vi "test TCX read (installed 71).vi"() -> ()   [LabVIEW 2011] (continued)
rees></Position><AltitudeMeters>71.275</AltitudeMeters><DistanceMeters>20043.990</DistanceMeters><Cadence>68</Cadence><Extensions><TPX xmlns=\"http://www.garmin.com/xmlschemas/ActivityExtension/v2\"><Watts>169</Watts></TPX></Extensions></Trackpoint><Trackpoint><Time>2008-03-03T23:21:45Z</Time><Position><LatitudeDegrees>35.876197</LatitudeDegrees><LongitudeDegrees>-78.946791</LongitudeDegrees></Position><AltitudeMeters>71.755</AltitudeMeters><DistanceMeters>20051.418</DistanceMeters><Cadence>67</Cadence><Extensions><TPX xmlns=\"http://www.garmin.com/xmlschemas/ActivityExtension/v2\"><Watts>175</Watts></TPX></Extensions></Trackpoint><Trackpoint><Time>2008-03-03T23:21:46Z</Time><Position><LatitudeDegrees>35.876203</LatitudeDegrees><LongitudeDegrees>-78.946872</LongitudeDegrees></Position><AltitudeMeters>72.236</AltitudeMeters><DistanceMeters>20058.742</DistanceMeters><Cadence>67</Cadence><Extensions><TPX xmlns=\"http://www.garmin.com/xmlschemas/ActivityExtension/v2\"><Watts>174</Watts></TPX></Extensions></Trackpoint><Trackpoint><Time>2008-03-03T23:21:47Z</Time><Position><LatitudeDegrees>35.876206</LatitudeDegrees><LongitudeDegrees>-78.946951</LongitudeDegrees></Position><AltitudeMeters>72.236</AltitudeMeters><DistanceMeters>20065.842</DistanceMeters><Cadence>65</Cadence><Extensions><TPX xmlns=\"http://www.garmin.com/xmlschemas/ActivityExtension/v2\"><Watts>166</Watts></TPX></Extensions></Trackpoint><Trackpoint><Time>2008-03-03T23:21:48Z</Time><Position><LatitudeDegrees>35.876207</LatitudeDegrees><LongitudeDegrees>-78.947027</LongitudeDegrees></Position><AltitudeMeters>72.236</AltitudeMeters><DistanceMeters>20072.709</DistanceMeters><Cadence>63</Cadence><Extensions><TPX xmlns=\"http://www.garmin.com/xmlschemas/ActivityExtension/v2\"><Watts>171</Watts></TPX></Extensions></Trackpoint><Trackpoint><Time>2008-03-03T23:21:49Z</Time><Position><LatitudeDegrees>35.876210</LatitudeDegrees><LongitudeDegrees>-78.947102</LongitudeDegrees></Position><AltitudeMeters>72.236</AltitudeMeters><DistanceMeters>20079.447</DistanceMeters><Cadence>62</Cadence><Extensions><TPX xmlns=\"http://www.garmin.com/xmlschemas/ActivityExtension/v2\"><Watts>177</Watts></TPX></Extensions></Trackpoint><Trackpoint><Time>2008-03-03T23:21:50Z</Time><Position><LatitudeDegrees>35.876215</LatitudeDegrees><LongitudeDegrees>-78.947175</LongitudeDegrees></Position><AltitudeMeters>72.717</AltitudeMeters><DistanceMeters>20086.098</DistanceMeters><Cadence>68</Cadence><Extensions><TPX xmlns=\"http://www.garmin.com/xmlschemas/ActivityExtension/v2\"><Watts>192</Watts></TPX></Extensions></Trackpoint><Trackpoint><Time>2008-03-03T23:21:51Z</Time><Position><LatitudeDegrees>35.876220</LatitudeDegrees><LongitudeDegrees>-78.947248</LongitudeDegrees></Position><AltitudeMeters>72.717</AltitudeMeters><DistanceMeters>20092.703</DistanceMeters><Cadence>68</Cadence><Extensions><TPX xmlns=\"http://www.garmin.com/xmlschemas/ActivityExtension/v2\"><Watts>200</Watts></TPX></Extensions></Trackpoint><Trackpoint><Time>2008-03-03T23:21:52Z</Time><Position><LatitudeDegrees>35.876223</LatitudeDegrees><LongitudeDegrees>-78.947321</LongitudeDegrees></Position><AltitudeMeters>73.198</AltitudeMeters><DistanceMeters>20099.342</DistanceMeters><Cadence>68</Cadence><Extensions><TPX xmlns=\"http://www.garmin.com/xmlschemas/ActivityExtension/v2\"><Watts>201</Watts></TPX></Extensions></Trackpoint><Trackpoint><Time>2008-03-03T23:21:53Z</Time><Position><LatitudeDegrees>35.876227</LatitudeDegrees><LongitudeDegrees>-78.947395</LongitudeDegrees></Position><AltitudeMeters>73.198</AltitudeMeters><DistanceMeters>20106.008</DistanceMeters><Cadence>67</Cadence><Extensions><TPX xmlns=\"http://www.garmin.com/xmlschemas/ActivityExtension/v2\"><Watts>197</Watts></TPX></Extensions></Trackpoint><Trackpoint><Time>2008-03-03T23:21:54Z</Time><Position><LatitudeDegrees>35.876231</LatitudeDegrees><LongitudeDegrees>-78.947468</LongitudeDegrees></Position><AltitudeMeters>73.198</AltitudeMeters><DistanceMeters>20112.586</DistanceMeters><Cadence>67</Cadence><Extensions><TPX xmlns=\"http://www.garmin.com/xmlschemas/ActivityExtension/v2\"><Watts>192</Watts></TPX></Extensions></Trackpoint><Trackpoint><Time>2008-03-03T23:21:55Z</Time><Position><LatitudeDegrees>35.876232</LatitudeDegrees><LongitudeDegrees>-78.947539</LongitudeDegrees></Position><AltitudeMeters>73.198</AltitudeMeters><DistanceMeters>20118.984</DistanceMeters><Cadence>66</Cadence><Extensions><TPX xmlns=\"http://www.garmin.com/xmlschemas/ActivityExtension/v2\"><Watts>180</Watts></TPX></Extensions></Trackpoint><Trackpoint><Time>2008-03-03T23:21:56Z</Time><Position><LatitudeDegrees>35.876232</LatitudeDegrees><LongitudeDegrees>-78.947610</LongitudeDegrees></Position><AltitudeMeters>73.678</AltitudeMeters><DistanceMeters>20125.402</DistanceMeters><Cadence>66</Cadence><Extensions><TPX xmlns=\"http://www.garmin.com/xmlschemas/ActivityExtension/v2\"><Watts>188</Watts></TPX></Extensions></Trackpoint><Trackpoint><Time>2008-03-03T23:21:57Z</Time><Position><LatitudeDegrees>35.876234</LatitudeDegrees><LongitudeDegrees>-78.947681</LongitudeDegrees></Position><AltitudeMeters>73.678</AltitudeMeters><DistanceMeters>20131.861</DistanceMeters><Cadence>66</Cadence><Extensions><TPX xmlns=\"http://www.garmin.com/xmlschemas/ActivityExtension/v2\"><Watts>208</Watts></TPX></Extensions></Trackpoint><Trackpoint><Time>2008-03-03T23:21:58Z</Time><Position><LatitudeDegrees>35.876237</LatitudeDegrees><LongitudeDegrees>-78.947754</LongitudeDegrees></Position><AltitudeMeters>73.678</AltitudeMeters><DistanceMeters>20138.393</DistanceMeters><Cadence>67</Cadence><Extensions><TPX xmlns=\"http://www.garmin.com/xmlschemas/ActivityExtension/v2\"><Watts>229</Watts></TPX></Extensions></Trackpoint><Trackpoint><Time>2008-03-03T23:21:59Z</Time><Position><LatitudeDegrees>35.876237</LatitudeDegrees><LongitudeDegrees>-78.947827</LongitudeDegrees></Position><AltitudeMeters>74.159</AltitudeMeters><DistanceMeters>20145.053</DistanceMeters><Cadence>68</Cadence><Extensions><TPX xmlns=\"http://www.garmin.com/xmlschemas/ActivityExtension/v2\"><Watts>237</Watts></TPX></Extensions></Trackpoint><Trackpoint><Time>2008-03-03T23:22:00Z</Time><Position><LatitudeDegrees>35.876238</LatitudeDegrees><LongitudeDegrees>-78.947902</LongitudeDegrees></Position><AltitudeMeters>74.159</AltitudeMeters><DistanceMeters>20151.803</DistanceMeters><Cadence>70</Cadence><Extensions><TPX xmlns=\"http://www.garmin.com/xmlschemas/ActivityExtension/v2\"><Watts>248</Watts></TPX></Extensions></Trackpoint><Trackpoint><Time>2008-03-03T23:22:01Z</Time><Position><LatitudeDegrees>35.876241</LatitudeDegrees><LongitudeDegrees>-78.947977</LongitudeDegrees></Position><AltitudeMeters>74.640</AltitudeMeters><DistanceMeters>20158.611</DistanceMeters><Cadence>70</Cadence><Extensions><TPX xmlns=\"http://www.garmin.com/xmlschemas/ActivityExtension/v2\"><Watts>248</Watts></TPX></Extensions></Trackpoint><Trackpoint><Time>2008-03-03T23:22:02Z</Time><Position><LatitudeDegrees>35.876244</LatitudeDegrees><LongitudeDegrees>-78.948055</LongitudeDegrees></Position><AltitudeMeters>74.640</AltitudeMeters><DistanceMeters>20165.658</DistanceMeters><Cadence>73</Cadence><Extensions><TPX xmlns=\"http://www.garmin.com/xmlschemas/ActivityExtension/v2\"><Watts>331</Watts></TPX></Extensions></Trackpoint><Trackpoint><Time>2008-03-03T23:22:03Z</Time><Position><LatitudeDegrees>35.876247</LatitudeDegrees><LongitudeDegrees>-78.948135</LongitudeDegrees></Position><AltitudeMeters>74.640</AltitudeMeters><DistanceMeters>20172.889</DistanceMeters><Cadence>75</Cadence><Extensions><TPX xmlns=\"http://www.garmin.com/xmlschemas/ActivityExtension/v2\"><Watts>377</Watts></TPX></Extensions></Trackpoint><Trackpoint><Time>2008-03-03T23:22:04Z</Time><Position><LatitudeDegrees>35.876249</LatitudeDegrees><LongitudeDegrees>-78.948216</LongitudeDegrees></Position><AltitudeMeters>75.120</AltitudeMeters><DistanceMeters>20180.209</DistanceMeters><Cadence>75</Cadence><Extensions><TPX xmlns=\"http://www.garmin.com/xmlschemas/ActivityExtension/v2\"><Watts>376</Watts></TPX></Extensions></Trackpoint><Trackpoint><Time>2008-03-03T23:22:05Z</Time><Position><LatitudeDegrees>35.876251</LatitudeDegrees><LongitudeDegrees>-78.948297</LongitudeDegrees></Position><AltitudeMeters>75.120</AltitudeMeters><DistanceMeters>20187.525</DistanceMeters><Cadence>74</Cadence><Extensions><TPX xmlns=\"http://www.garmin.com/xmlschemas/ActivityExtension/v2\"><Watts>258</Watts></TPX></Extensions></Trackpoint><Trackpoint><Time>2008-03-03T23:22:06Z</Time><Position><LatitudeDegrees>35.876256</LatitudeDegrees><LongitudeDegrees>-78.948378</LongitudeDegrees></Position><AltitudeMeters>75.601</AltitudeMeters><DistanceMeters>20194.811</DistanceMeters><Cadence>74</Cadence><Extensions><TPX xmlns=\"http://www.garmin.com/xmlschemas/ActivityExtension/v2\"><Watts>259</Watts></TPX></Extensions></Trackpoint><Trackpoint><Time>2008-03-03T23:22:07Z</Time><Position><LatitudeDegrees>35.876258</LatitudeDegrees><LongitudeDegrees>-78.948457</LongitudeDegrees></Position><AltitudeMeters>75.601</AltitudeMeters><DistanceMeters>20201.953</DistanceMeters><Cadence>74</Cadence><Extensions><TPX xmlns=\"http://www.garmin.com/xmlschemas/ActivityExtension/v2\"><Watts>223</Watts></TPX></Extensions></Trackpoint><Trackpoint><Time>2008-03-03T23:22:08Z</Time><Position><LatitudeDegrees>35.876259</LatitudeDegrees><LongitudeDegrees>-78.948533</LongitudeDegrees></Position><AltitudeMeters>75.601</AltitudeMeters><DistanceMeters>20208.805</DistanceMeters><Cadence>71</Cadence><Extensions><TPX xmlns=\"http://www.garmin.com/xmlschemas/ActivityExtension/v2\"><Watts>199</Watts></TPX></Extensions></Trackpoint><Trackpoint><Time>2008-03-03T23:22:09Z</Time><Position><LatitudeDegrees>35.876260</LatitudeDegrees><LongitudeDegrees>-78.948607</LongitudeDegrees></Position><AltitudeMeters>75.601</AltitudeMeters><DistanceMeters>20215.475</DistanceMeters><Cadence>69</Cadence><Extensions><TPX xmlns=\"http://www.garmin.com/xmlschemas/ActivityExtension/v2\"><Watts>153</Watts></TPX></Extensions></Trackpoint><Trackpoint><Time>2008-03-03T23:22:10Z</Time><Position><LatitudeDegrees>35.876262</LatitudeDegrees><LongitudeDegrees>-78.948679</LongitudeDegrees></Position><AltitudeMeters>75.601</AltitudeMeters><DistanceMeters>20221.939</DistanceMeters><Cadence>67</Cadence><Extensions><TPX xmlns=\"http://www.garmin.com/xmlschemas/ActivityExtension/v2\"><Watts>99</Watts></TPX></Extensions></Trackpoint><Trackpoint><Time>2008-03-03T23:22:11Z</Time><Position><LatitudeDegrees>35.876262</LatitudeDegrees><LongitudeDegrees>-78.948745</LongitudeDegrees></Position><AltitudeMeters>76.081</AltitudeMeters><DistanceMeters>20227.865</DistanceMeters><Cadence>67</Cadence><Extensions><TPX xmlns=\"http://www.garmin.com/xmlschemas/ActivityExtension/v2\"><Watts>100</Watts></TPX></Extensions></Trackpoint><Trackpoint><Time>2008-03-03T23:22:12Z</Time><Position><LatitudeDegrees>35.876267</LatitudeDegrees><LongitudeDegrees>-78.948802</LongitudeDegrees></Position><AltitudeMeters>76.081</AltitudeMeters><DistanceMeters>20233.020</DistanceMeters><Cadence>27</Cadence><Extensions><TPX xmlns=\"http://www.garmin.com/xmlschemas/ActivityExtension/v2\"><Watts>52</Watts></TPX></Extensions></Trackpoint><Trackpoint><Time>2008-03-03T23:22:13Z</Time><Position><LatitudeDegrees>35.876282</LatitudeDegrees><LongitudeDegrees>-78.948850</LongitudeDegrees></Position><AltitudeMeters>76.081</AltitudeMeters><DistanceMeters>20237.607</DistanceMeters><Cadence>27</Cadence><Extensions><TPX xmlns=\"http://www.garmin.com/xmlschemas/ActivityExtension/v2\"><Watts>52</Watts></TPX></Extensions></Trackpoint><Trackpoint><Time>2008-03-03T23:22:14Z</Time><Position><LatitudeDegrees>35.876308</LatitudeDegrees><LongitudeDegrees>-78.948884</LongitudeDegrees></Position><AltitudeMeters>76.562</AltitudeMeters><DistanceMeters>20241.734</DistanceMeters><Cadence>50</Cadence><Extensions><TPX xmlns=\"http://www.garmin.com/xmlschemas/ActivityExtension/v2\"><Watts>129</Watts></TPX></Extensions></Trackpoint><Trackpoint><Time>2008-03-03T23:22:15Z</Time><Position><LatitudeDegrees>35.876342</LatitudeDegrees><LongitudeDegrees>-78.948896</LongitudeDegrees></Position><AltitudeMeters>76.081</AltitudeMeters><DistanceMeters>20245.682</DistanceMeters><Cadence>55</Cadence><Extensions><TPX xmlns=\"http://www.garmin.com/xmlschemas/ActivityExtension/v2\"><Watts>154</Watts></TPX></Extensions></Trackpoint><Trackpoint><Time>2008-03-03T23:22:16Z</Time><Position><LatitudeDegrees>35.876388</LatitudeDegrees><LongitudeDegrees>-78.948887</LongitudeDegrees></Position><AltitudeMeters>75.601</AltitudeMeters><DistanceMeters>20250.920</DistanceMeters><Cadence>55</Cadence><Extensions><TPX xmlns=\"http://www.garmin.com/xmlschemas/ActivityExtension/v2\"><Watts>153</Watts></TPX></Extensions></Trackpoint><Trackpoint><Time>2008-03-03T23:22:17Z</Time><Position><LatitudeDegrees>35.876442</LatitudeDegrees><LongitudeDegrees>-78.948871</LongitudeDegrees></Position><AltitudeMeters>75.601</AltitudeMeters><DistanceMeters>20257.107</DistanceMeters><Cadence>66</Cadence><Extensions><TPX xmlns=\"http://www.garmin.com/xmlschemas/ActivityExtension/v2\"><Watts>222</Watts></TPX></Extensions></Trackpoint><Trackpoint><Time>2008-03-03T23:22:18Z</Time><Position><LatitudeDegrees>35.876501</LatitudeDegrees><LongitudeDegrees>-78.948851</LongitudeDegrees></Position><AltitudeMeters>75.601</AltitudeMeters><DistanceMeters>20263.939</DistanceMeters><Cadence>66</Cadence><Extensions><TPX xmlns=\"http://www.garmin.com/xmlschemas/ActivityExtension/v2\"><Watts>223</Watts></TPX></Extensions></Trackpoint><Trackpoint><Time>2008-03-03T23:22:19Z</Time><Position><LatitudeDegrees>35.876563</LatitudeDegrees><LongitudeDegrees>-78.948830</LongitudeDegrees></Position><AltitudeMeters>75.120</AltitudeMeters><DistanceMeters>20271.023</DistanceMeters><Cadence>66</Cadence><Extensions><TPX xmlns=\"http://www.garmin.com/xmlschemas/ActivityExtension/v2\"><Watts>214</Watts></TPX></Extensions></Trackpoint><Trackpoint><Time>2008-03-03T23:22:20Z</Time><Position><LatitudeDegrees>35.876627</LatitudeDegrees><LongitudeDegrees>-78.948809</LongitudeDegrees></Position><AltitudeMeters>75.601</AltitudeMeters><DistanceMeters>20278.404</DistanceMeters><Cadence>69</Cadence><Extensions><TPX xmlns=\"http://www.garmin.com/xmlschemas/ActivityExtension/v2\"><Watts>186</Watts></TPX></Extensions></Trackpoint><Trackpoint><Time>2008-03-03T23:22:21Z</Time><Position><LatitudeDegrees>35.876695</LatitudeDegrees><LongitudeDegrees>-78.948788</LongitudeDegrees></Position><AltitudeMeters>75.120</AltitudeMeters><DistanceMeters>20286.246</DistanceMeters><Cadence>72</Cadence><Extensions><TPX xmlns=\"http://www.garmin.com/xmlschemas/ActivityExtension/v2\"><Watts>186</Watts></TPX></Extensions></Trackpoint><Trackpoint><Time>2008-03-03T23:22:22Z</Time><Position><LatitudeDegrees>35.876768</LatitudeDegrees><LongitudeDegrees>-78.948767</LongitudeDegrees></Position><AltitudeMeters>75.120</AltitudeMeters><DistanceMeters>20294.619</DistanceMeters><Cadence>79</Cadence><Extensions><TPX xmlns=\"http://www.garmin.com/xmlschemas/ActivityExtension/v2\"><Watts>217</Watts></TPX></Extensions></Trackpoint><Trackpoint><Time>2008-03-03T23:22:23Z</Time><Position><LatitudeDegrees>35.876845</LatitudeDegrees><LongitudeDegrees>-78.948744</LongitudeDegrees></Position><AltitudeMeters>75.120</AltitudeMeters><DistanceMeters>20303.367</DistanceMeters><Cadence>79</Cadence><Extensions><TPX xmlns=\"http://www.garmin.com/xmlschemas/ActivityExtension/v2\"><Watts>232</Watts></TPX></Extensions></Trackpoint><Trackpoint><Time>2008-03-03T23:22:24Z</Time><Position><LatitudeDegrees>35.876926</LatitudeDegrees><LongitudeDegrees>-78.948722</LongitudeDegrees></Position><AltitudeMeters>75.120</AltitudeMeters><DistanceMeters>20312.650</DistanceMeters><Cadence>87</Cadence><Extensions><TPX xmlns=\"http://www.garmin.com/xmlschemas/ActivityExtension/v2\"><Watts>318</Watts></TPX></Extensions></Trackpoint><Trackpoint><Time>2008-03-03T23:22:25Z</Time><Position><LatitudeDegrees>35.877009</LatitudeDegrees><LongitudeDegrees>-78.948700</LongitudeDegrees></Position><AltitudeMeters>75.601</AltitudeMeters><DistanceMeters>20322.072</DistanceMeters><Cadence>87</Cadence><Extensions><TPX xmlns=\"http://www.garmin.com/xmlschemas/ActivityExtension/v2\"><Watts>321</Watts></TPX></Extensions></Trackpoint><Trackpoint><Time>2008-03-03T23:22:26Z</Time><Position><LatitudeDegrees>35.877106</LatitudeDegrees><LongitudeDegrees>-78.948673</LongitudeDegrees></Position><AltitudeMeters>75.601</AltitudeMeters><DistanceMeters>20333.141</DistanceMeters><Cadence>88</Cadence><Extensions><TPX xmlns=\"http://www.garmin.com/xmlschemas/ActivityExtension/v2\"><Watts>142</Watts></TPX></Extensions></Trackpoint><Trackpoint><Time>2008-03-03T23:22:27Z</Time><Position><LatitudeDegrees>35.877202</LatitudeDegrees><LongitudeDegrees>-78.948628</LongitudeDegrees></Position><AltitudeMeters>75.601</AltitudeMeters><DistanceMeters>20344.402</DistanceMeters><Cadence>89</Cadence><Extensions><TPX xmlns=\"http://www.garmin.com/xmlschemas/ActivityExtension/v2\"><Watts>132</Watts></TPX></Extensions></Trackpoint><Trackpoint><Time>2008-03-03T23:22:28Z</Time><Position><LatitudeDegrees>35.877294</LatitudeDegrees><LongitudeDegrees>-78.948611</LongitudeDegrees></Position><AltitudeMeters>75.601</AltitudeMeters><DistanceMeters>20354.625</DistanceMeters><Cadence>89</Cadence><Extensions><TPX xmlns=\"http://www.garmin.com/xmlschemas/ActivityExtension/v2\"><Watts>131</Watts></TPX></Extensions></Trackpoint><Trackpoint><Time>2008-03-03T23:22:29Z</Time><Position><LatitudeDegrees>35.877387</LatitudeDegrees><LongitudeDegrees>-78.948580</LongitudeDegrees></Position><AltitudeMeters>75.601</AltitudeMeters><DistanceMeters>20365.342</DistanceMeters><Cadence>90</Cadence><Extensions><TPX xmlns=\"http://www.garmin.com/xmlschemas/ActivityExtension/v2\"><Watts>142</Watts></TPX></Extensions></Trackpoint><Trackpoint><Time>2008-03-03T23:22:30Z</Time><Position><LatitudeDegrees>35.877478</LatitudeDegrees><LongitudeDegrees>-78.948560</LongitudeDegrees></Position><AltitudeMeters>75.601</AltitudeMeters><DistanceMeters>20375.645</DistanceMeters><Cadence>90</Cadence><Extensions><TPX xmlns=\"http://www.garmin.com/xmlschemas/ActivityExtension/v2\"><Watts>137</Watts></TPX></Extensions></Trackpoint><Trackpoint><Time>2008-03-03T23:22:31Z</Time><Position><LatitudeDegrees>35.877568</LatitudeDegrees><LongitudeDegrees>-78.948537</LongitudeDegrees></Position><AltitudeMeters>74.640</AltitudeMeters><DistanceMeters>20385.846</DistanceMeters><Cadence>90</Cadence><Extensions><TPX xmlns=\"http://www.garmin.com/xmlschemas/ActivityExtension/v2\"><Watts>138</Watts></TPX></Extensions></Trackpoint><Trackpoint><Time>2008-03-03T23:22:32Z</Time><Position><LatitudeDegrees>35.877655</LatitudeDegrees><LongitudeDegrees>-78.948516</LongitudeDegrees></Position><AltitudeMeters>75.120</AltitudeMeters><DistanceMeters>20395.629</DistanceMeters><Cadence>92</Cadence><Extensions><TPX xmlns=\"http://www.garmin.com/xmlschemas/ActivityExtension/v2\"><Watts>132</Watts></TPX></Extensions></Trackpoint><Trackpoint><Time>2008-03-03T23:22:33Z</Time><Position><LatitudeDegrees>35.877741</LatitudeDegrees><LongitudeDegrees>-78.948493</LongitudeDegrees></Position><AltitudeMeters>75.120</AltitudeMeters><DistanceMeters>20405.471</DistanceMeters><Cadence>92</Cadence><Extensions><TPX xmlns=\"http://www.garmin.com/xmlschemas/ActivityExtension/v2\"><Watts>132</Watts></TPX></Extensions></Trackpoint><Trackpoint><Time>2008-03-03T23:22:34Z</Time><Position><LatitudeDegrees>35.877831</LatitudeDegrees><LongitudeDegrees>-78.948470</LongitudeDegrees></Position><AltitudeMeters>74.640</AltitudeMeters><DistanceMeters>20415.629</DistanceMeters><Cadence>93</Cadence><Extensions><TPX xmlns=\"http://www.garmin.com/xmlschemas/ActivityExtension/v2\"><Watts>154</Watts></TPX></Extensions></Trackpoint><Trackpoint><Time>2008-03-03T23:22:35Z</Time><Position><LatitudeDegrees>35.877921</LatitudeDegrees><LongitudeDegrees>-78.948445</LongitudeDegrees></Position><AltitudeMeters>75.120</AltitudeMeters><DistanceMeters>20425.867</DistanceMeters><Cadence>93</Cadence><Extensions><TPX xmlns=\"http://www.garmin.com/xmlschemas/ActivityExtension/v2\"><Watts>153</Watts></TPX></Extensions></Trackpoint><Trackpoint><Time>2008-03-03T23:22:36Z</Time><Position><LatitudeDegrees>35.878009</LatitudeDegrees><LongitudeDegrees>-78.948421</LongitudeDegrees></Position><AltitudeMeters>75.120</AltitudeMeters><DistanceMeters>20435.811</DistanceMeters><Cadence>93</Cadence><Extensions><TPX xmlns=\"http://www.garmin.com/xmlschemas/ActivityExtension/v2\"><Watts>114</Watts></TPX></Extensions></Trackpoint><Trackpoint><Time>2008-03-03T23:22:37Z</Time><Position><LatitudeDegrees>35.878098</LatitudeDegrees><LongitudeDegrees>-78.948397</LongitudeDegrees></Position><AltitudeMeters>74.159</AltitudeMeters><DistanceMeters>20445.957</DistanceMeters><Cadence>93</Cadence><Extensions><TPX xmlns=\"http://www.garmin.com/xmlschemas/ActivityExtension/v2\"><Watts>99</Watts></TPX></Extensions></Trackpoint><Trackpoint><Time>2008-03-03T23:22:38Z</Time><Position><LatitudeDegrees>35.878186</LatitudeDegrees><LongitudeDegrees>-78.948375</LongitudeDegrees></Position><AltitudeMeters>74.159</AltitudeMeters><DistanceMeters>20455.955</DistanceMeters><Cadence>93</Cadence><Extensions><TPX xmlns=\"http://www.garmin.com/xmlschemas/ActivityExtension/v2\"><Watts>97</Watts></TPX></Extensions></Trackpoint><Trackpoint><Time>2008-03-03T23:22:39Z</Time><Position><LatitudeDegrees>35.878275</LatitudeDegrees><LongitudeDegrees>-78.948352</LongitudeDegrees></Position><AltitudeMeters>74.159</AltitudeMeters><DistanceMeters>20466.039</DistanceMeters><Cadence>93</Cadence><Extensions><TPX xmlns=\"http://www.garmin.com/xmlschemas/ActivityExtension/v2\"><Watts>99</Watts></TPX></Extensions></Trackpoint><Trackpoint><Time>2008-03-03T23:22:40Z</Time><Position><LatitudeDegrees>35.878364</LatitudeDegrees><LongitudeDegrees>-78.948330</LongitudeDegrees></Position><AltitudeMeters>74.159</AltitudeMeters><DistanceMeters>20476.113</DistanceMeters><Cadence>93</Cadence><Extensions><TPX xmlns=\"http://www.garmin.com/xmlschemas/ActivityExtension/v2\"><Watts>95</Watts></TPX></Extensions></Trackpoint><Trackpoint><Time>2008-03-03T23:22:41Z</Time><Position><LatitudeDegrees>35.878452</LatitudeDegrees><LongitudeDegrees>-78.948306</LongitudeDegrees></Position><AltitudeMeters>74.159</AltitudeMeters><DistanceMeters>20486.135</DistanceMeters><Cadence>93</Cadence><Extensions><TPX xmlns=\"http://www.garmin.com/xmlschemas/ActivityExtension/v2\"><Watts>94</Watts></TPX></Extensions></Trackpoint><Trackpoint><Time>2008-03-03T23:22:42Z</Time><Position><LatitudeDegrees>35.878541</LatitudeDegrees><LongitudeDegrees>-78.948282</LongitudeDegrees></Position><AltitudeMeters>74.159</AltitudeMeters><DistanceMeters>20496.225</DistanceMeters><Cadence>94</Cadence><Extensions><TPX xmlns=\"http://www.garmin.com/xmlschemas/ActivityExtension/v2\"><Watts>113</Watts></TPX></Extensions></Trackpoint><Trackpoint><Time>2008-03-03T23:22:43Z</Time><Position><LatitudeDegrees>35.878631</LatitudeDegrees><LongitudeDegrees>-78.948260</LongitudeDegrees></Position><AltitudeMeters>74.159</AltitudeMeters><DistanceMeters>20506.412</DistanceMeters><Cadence>94</Cadence><Extensions><TPX xmlns=\"http://www.garmin.com/xmlschemas/ActivityExtension/v2\"><Watts>113</Watts></TPX></Extensions></Trackpoint><Trackpoint><Time>2008-03-03T23:22:44Z</Time><Position><LatitudeDegrees>35.878723</LatitudeDegrees><LongitudeDegrees>-78.948236</LongitudeDegrees></Position><AltitudeMeters>74.159</AltitudeMeters><DistanceMeters>20516.883</DistanceMeters><Cadence>98</Cadence><Extensions><TPX xmlns=\"http://www.garmin.com/xmlschemas/ActivityExtension/v2\"><Watts>291</Watts></TPX></Extensions></Trackpoint><Trackpoint><Time>2008-03-03T23:22:45Z</Time><Position><LatitudeDegrees>35.878816</LatitudeDegrees><LongitudeDegrees>-78.948210</LongitudeDegrees></Position><AltitudeMeters>73.678</AltitudeMeters><DistanceMeters>20527.412</DistanceMeters><Cadence>99</Cadence><Extensions><TPX xmlns=\"http://www.garmin.com/xmlschemas/ActivityExtension/v2\"><Watts>295</Watts></TPX></Extensions></Trackpoint><Trackpoint><Time>2008-03-03T23:22:46Z</Time><Position><LatitudeDegrees>35.878911</LatitudeDegrees><LongitudeDegrees>-78.948183</LongitudeDegrees></Position><AltitudeMeters>74.159</AltitudeMeters><DistanceMeters>20538.232</DistanceMeters><Cadence>98</Cadence><Extensions><TPX xmlns=\"http://www.garmin.com/xmlschemas/ActivityExtension/v2\"><Watts>193</Watts></TPX></Extensions></Trackpoint><Trackpoint><Time>2008-03-03T23:22:47Z</Time><Position><LatitudeDegrees>35.879006</LatitudeDegrees><LongitudeDegrees>-78.948157</LongitudeDegrees></Position><AltitudeMeters>74.159</AltitudeMeters><DistanceMeters>20549.020</DistanceMeters><Cadence>98</Cadence><Extensions><TPX xmlns=\"http://www.garmin.com/xmlschemas/ActivityExtension/v2\"><Watts>150</Watts></TPX></Extensions></Trackpoint><Trackpoint><Time>2008-03-03T23:22:48Z</Time><Position><LatitudeDegrees>35.879100</LatitudeDegrees><LongitudeDegrees>-78.948131</LongitudeDegrees></Position><AltitudeMeters>74.159</AltitudeMeters><DistanceMeters>20559.719</DistanceMeters><Cadence>98</Cadence><Extensions><TPX xmlns=\"http://www.garmin.com/xmlschemas/ActivityExtension/v2\"><Watts>148</Watts></TPX></Extensions></Trackpoint><Trackpoint><Time>2008-03-03T23:22:49Z</Time><Position><LatitudeDegrees>35.879193</LatitudeDegrees><LongitudeDegrees>-78.948105</LongitudeDegrees></Position><AltitudeMeters>74.159</AltitudeMeters><DistanceMeters>20570.318</DistanceMeters><Cadence>98</Cadence><Extensions><TPX xmlns=\"http://www.garmin.com/xmlschemas/ActivityExtension/v2\"><Watts>138</Watts></TPX></Extensions></Trackpoint><Trackpoint><Time>2008-03-03T23:22:50Z</Time><Position><LatitudeDegrees>35.879288</LatitudeDegrees><LongitudeDegrees>-78.948090</LongitudeDegrees></Position><AltitudeMeters>74.640</AltitudeMeters><DistanceMeters>20580.850</DistanceMeters><Cadence>96</Cadence><Extensions><TPX xmlns=\"http://www.garmin.com/xmlschemas/ActivityExtension/v2\"><Watts>129</Watts></TPX></Extensions></Trackpoint><Trackpoint><Time>2008-03-03T23:22:51Z</Time><Position><LatitudeDegrees>35.879378</LatitudeDegrees><LongitudeDegrees>-78.948067</LongitudeDegrees></Position><AltitudeMeters>74.640</AltitudeMeters><DistanceMeters>20591.127</DistanceMeters><Cadence>93</Cadence><Extensions><TPX xmlns=\"http://www.garmin.com/xmlschemas/ActivityExtension/v2\"><Watts>122</Watts></TPX></Extensions></Trackpoint><Trackpoint><Time>2008-03-03T23:22:52Z</Time><Position><LatitudeDegrees>35.879468</LatitudeDegrees><LongitudeDegrees>-78.948041</LongitudeDegrees></Position><AltitudeMeters>75.120</AltitudeMeters><DistanceMeters>20601.312</DistanceMeters><Cadence>92</Cadence><Extensions><TPX xmlns=\"http://www.garmin.com/xmlschemas/ActivityExtension/v2\"><Watts>121</Watts></TPX></Extensions></Trackpoint><Trackpoint><Time>2008-03-03T23:22:53Z</Time><Position><LatitudeDegrees>35.879554</LatitudeDegrees><LongitudeDegrees>-78.948017</LongitudeDegrees></Position><AltitudeMeters>74.640</AltitudeMeters><DistanceMeters>20611.094</DistanceMeters><Cadence>91</Cadence><Extensions><TPX xmlns=\"http://www.garmin.com/xmlschemas/ActivityExtension/v2\"><Watts>118</Watts></TPX></Extensions></Trackpoint><Trackpoint><Time>2008-03-03T23:22:54Z</Time><Position><LatitudeDegrees>35.879638</LatitudeDegrees><LongitudeDegrees>-78.947994</LongitudeDegrees></Position><AltitudeMeters>75.120</AltitudeMeters><DistanceMeters>20620.662</DistanceMeters><Cadence>88</Cadence><Extensions><TPX xmlns=\"http://www.garmin.com/xmlschemas/ActivityExtension/v2\"><Watts>110</Watts></TPX></Extensions></Trackpoint><Trackpoint><Time>2008-03-03T23:22:55Z</Time><Position><LatitudeDegrees>35.879718</LatitudeDegrees><LongitudeDegrees>-78.947971</LongitudeDegrees></Position><AltitudeMeters>74.640</AltitudeMeters><DistanceMeters>20629.770</DistanceMeters><Cadence>86</Cadence><Extensions><TPX xmlns=\"http://www.garmin.com/xmlschemas/ActivityExtension/v2\"><Watts>110</Watts></TPX></Extensions></Trackpoint><Trackpoint><Time>2008-03-03T23:22:56Z</Time><Position><LatitudeDegrees>35.879798</LatitudeDegrees><LongitudeDegrees>-78.947949</LongitudeDegrees></Position><AltitudeMeters>74.640</AltitudeMeters><DistanceMeters>20638.779</DistanceMeters><Cadence>84</Cadence><Extensions><TPX xmlns=\"http://www.garmin.com/xmlschemas/ActivityExtension/v2\"><Watts>114</Watts></TPX></Extensions></Trackpoint><Trackpoint><Time>2008-03-03T23:22:57Z</Time><Position><LatitudeDegrees>35.879876</LatitudeDegrees><LongitudeDegrees>-78.947927</LongitudeDegrees></Position><AltitudeMeters>75.601</AltitudeMeters><DistanceMeters>20647.670</DistanceMeters><Cadence>83</Cadence><Extensions><TPX xmlns=\"http://www.garmin.com/xmlschemas/ActivityExtension/v2\"><Watts>118</Watts></TPX></Extensions></Trackpoint><Trackpoint><Time>2008-03-03T23:22:58Z</Time><Position><LatitudeDegrees>35.879953</LatitudeDegrees><LongitudeDegrees>-78.947906</LongitudeDegrees></Position><AltitudeMeters>75.120</AltitudeMeters><DistanceMeters>20656.467</DistanceMeters><Cadence>82</Cadence><Extensions><TPX xmlns=\"http://www.garmin.com/xmlschemas/ActivityExtension/v2\"><Watts>123</Watts></TPX></Extensions></Trackpoint><Trackpoint><Time>2008-03-03T23:22:59Z</Time><Position><LatitudeDegrees>35.880031</LatitudeDegrees><LongitudeDegrees>-78.947884</LongitudeDegrees></Position><AltitudeMeters>75.601</AltitudeMeters><DistanceMeters>20665.312</DistanceMeters><Cadence>80</Cadence><Extensions><TPX xmlns=\"http://www.garmin.com/xmlschemas/ActivityExtension/v2\"><Watts>148</Watts></TPX></Extensions></Trackpoint><Trackpoint><Time>2008-03-03T23:23:00Z</Time><Position><LatitudeDegrees>35.880107</LatitudeDegrees><LongitudeDegrees>-78.947864</LongitudeDegrees></Position><AltitudeMeters>75.601</AltitudeMeters><DistanceMeters>20673.875</DistanceMeters><Cadence>80</Cadence><Extensions><TPX xmlns=\"http://www.garmin.com/xmlschemas/ActivityExtension/v2\"><Watts>149</Watts></TPX></Extensions></Trackpoint><Trackpoint><Time>2008-03-03T23:23:01Z</Time><Position><LatitudeDegrees>35.880184</LatitudeDegrees><LongitudeDegrees>-78.947843</LongitudeDegrees></Position><AltitudeMeters>76.081</AltitudeMeters><DistanceMeters>20682.633</DistanceMeters><Cadence>80</Cadence><Extensions><TPX xmlns=\"http://www.garmin.com/xmlschemas/ActivityExtension/v2\"><Watts>236</Watts></TPX></Extensions></Trackpoint><Trackpoint><Time>2008-03-03T23:23:02Z</Time><Position><LatitudeDegrees>35.880259</LatitudeDegrees><LongitudeDegrees>-78.947821</LongitudeDegrees></Position><AltitudeMeters>76.081</AltitudeMeters><DistanceMeters>20691.289</DistanceMeters><Cadence>80</Cadence><Extensions><TPX xmlns=\"http://www.garmin.com/xmlschemas/ActivityExtension/v2\"><Watts>235</Watts></TPX></Extensions></Trackpoint><Trackpoint><Time>2008-03-03T23:23:03Z</Time><Position><LatitudeDegrees>35.880333</LatitudeDegrees><LongitudeDegrees>-78.947800</LongitudeDegrees></Position><AltitudeMeters>76.081</AltitudeMeters><DistanceMeters>20699.709</DistanceMeters><Cadence>79</Cadence><Extensions><TPX xmlns=\"http://www.garmin.com/xmlschemas/ActivityExtension/v2\"><Watts>249</Watts></TPX></Extensions></Trackpoint><Trackpoint><Time>2008-03-03T23:23:04Z</Time><Position><LatitudeDegrees>35.880408</LatitudeDegrees><LongitudeDegrees>-78.947779</LongitudeDegrees></Position><AltitudeMeters>76.562</AltitudeMeters><DistanceMeters>20708.225</DistanceMeters><Cadence>79</Cadence><Extensions><TPX xmlns=\"http://www.garmin.com/xmlschemas/ActivityExtension/v2\"><Watts>292</Watts></TPX></Extensions></Trackpoint><Trackpoint><Time>2008-03-03T23:23:05Z</Time><Position><LatitudeDegrees>35.880482</LatitudeDegrees><LongitudeDegrees>-78.947757</LongitudeDegrees></Position><AltitudeMeters>76.562</AltitudeMeters><DistanceMeters>20716.604</DistanceMeters><Cadence>79</Cadence><Extensions><TPX xmlns=\"http://www.garmin.com/xmlschemas/ActivityExtension/v2\"><Watts>290</Watts></TPX></Extensions></Trackpoint><Trackpoint><Time>2008-03-03T23:23:06Z</Time><Position><LatitudeDegrees>35.880556</LatitudeDegrees><LongitudeDegrees>-78.947735</LongitudeDegrees></Position><AltitudeMeters>76.562</AltitudeMeters><DistanceMeters>20725.094</DistanceMeters><Cadence>79</Cadence><Extensions><TPX xmlns=\"http://www.garmin.com/xmlschemas/ActivityExtension/v2\"><Watts>310</Watts></TPX></Extensions></Trackpoint><Trackpoint><Time>2008-03-03T23:23:07Z</Time><Position><LatitudeDegrees>35.880631</LatitudeDegrees><LongitudeDegrees>-78.947714</LongitudeDegrees></Position><AltitudeMeters>77.043</AltitudeMeters><DistanceMeters>20733.648</DistanceMeters><Cadence>79</Cadence><Extensions><TPX xmlns=\"http://www.garmin.com/xmlschemas/ActivityExtension/v2\"><Watts>298</Watts></TPX></Extensions></Trackpoint><Trackpoint><Time>2008-03-03T23:23:08Z</Time><Position><LatitudeDegrees>35.880707</LatitudeDegrees><LongitudeDegrees>-78.947692</LongitudeDegrees></Position><AltitudeMeters>77.043</AltitudeMeters><DistanceMeters>20742.355</DistanceMeters><Cadence>79</Cadence><Extensions><TPX xmlns=\"http://www.garmin.com/xmlschemas/ActivityExtension/v2\"><Watts>296</Watts></TPX></Extensions></Trackpoint><Trackpoint><Time>2008-03-03T23:23:09Z</Time><Position><LatitudeDegrees>35.880781</LatitudeDegrees><LongitudeDegrees>-78.947673</LongitudeDegrees></Position><AltitudeMeters>77.043</AltitudeMeters><DistanceMeters>20750.695</DistanceMeters><Cadence>78</Cadence><Extensions><TPX xmlns=\"http://www.garmin.com/xmlschemas/ActivityExtension/v2\"><Watts>285</Watts></TPX></Extensions></Trackpoint><Trackpoint><Time>2008-03-03T23:23:10Z</Time><Position><LatitudeDegrees>35.880856</LatitudeDegrees><LongitudeDegrees>-78.947657</LongitudeDegrees></Position><AltitudeMeters>77.043</AltitudeMeters><DistanceMeters>20759.082</DistanceMeters><Cadence>78</Cadence><Extensions><TPX xmlns=\"http://www.garmin.com/xmlschemas/ActivityExtension/v2\"><Watts>282</Watts></TPX></Extensions></Trackpoint><Trackpoint><Time>2008-03-03T23:23:11Z</Time><Position><LatitudeDegrees>35.880929</LatitudeDegrees><LongitudeDegrees>-78.947642</LongitudeDegrees></Position><AltitudeMeters>77.523</AltitudeMeters><DistanceMeters>20767.365</DistanceMeters><Cadence>77</Cadence><Extensions><TPX xmlns=\"http://www.garmin.com/xmlschemas/ActivityExtension/v2\"><Watts>201</Watts></TPX></Extensions></Trackpoint><Trackpoint><Time>2008-03-03T23:23:12Z</Time><Position><LatitudeDegrees>35.881002</LatitudeDegrees><LongitudeDegrees>-78.947626</LongitudeDegrees></Position><AltitudeMeters>77.523</AltitudeMeters><DistanceMeters>20775.592</DistanceMeters><Cadence>77</Cadence><Extensions><TPX xmlns=\"http://www.garmin.com/xmlschemas/ActivityExtension/v2\"><Watts>200</Watts></TPX></Extensions></Trackpoint><Trackpoint><Time>2008-03-03T23:23:13Z</Time><Position><LatitudeDegrees>35.881074</LatitudeDegrees><LongitudeDegrees>-78.947605</LongitudeDegrees></Position><AltitudeMeters>78.004</AltitudeMeters><DistanceMeters>20783.760</DistanceMeters><Cadence>76</Cadence><Extensions><TPX xmlns=\"http://www.garmin.com/xmlschemas/ActivityExtension/v2\"><Watts>195</Watts></TPX></Extensions></Trackpoint><Trackpoint><Time>2008-03-03T23:23:14Z</Time><Position><LatitudeDegrees>35.881145</LatitudeDegrees><LongitudeDegrees>-78.947582</LongitudeDegrees></Position><AltitudeMeters>78.004</AltitudeMeters><DistanceMeters>20791.947</DistanceMeters><Cadence>76</Cadence><Extensions><TPX xmlns=\"http://www.garmin.com/xmlschemas/ActivityExtension/v2\"><Watts>193</Watts></TPX></Extensions></Trackpoint><Trackpoint><Time>2008-03-03T23:23:15Z</Time><Position><LatitudeDegrees>35.881216</LatitudeDegrees><LongitudeDegrees>-78.947558</LongitudeDegrees></Position><AltitudeMeters>78.004</AltitudeMeters><DistanceMeters>20800.117</DistanceMeters><Cadence>76</Cadence><Extensions><TPX xmlns=\"http://www.garmin.com/xmlschemas/ActivityExtension/v2\"><Watts>215</Watts></TPX></Extensions></Trackpoint><Trackpoint><Time>2008-03-03T23:23:16Z</Time><Position><LatitudeDegrees>35.881288</LatitudeDegrees><LongitudeDegrees>-78.947533</LongitudeDegrees></Position><AltitudeMeters>78.004</AltitudeMeters><DistanceMeters>20808.332</DistanceMeters><Cadence>76</Cadence><Extensions><TPX xmlns=\"http://www.garmin.com/xmlschemas/ActivityExtension/v2\"><Watts>255</Watts></TPX></Extensions></Trackpoint><Trackpoint><Time>2008-03-03T23:23:17Z</Time><Position><LatitudeDegrees>35.881362</LatitudeDegrees><LongitudeDegrees>-78.947511</LongitudeDegrees></Position><AltitudeMeters>78.004</AltitudeMeters><DistanceMeters>20816.857</DistanceMeters><Cadence>79</Cadence><Extensions><TPX xmlns=\"http://www.garmin.com/xmlschemas/ActivityExtension/v2\"><Watts>316</Watts></TPX></Extensions></Trackpoint><Trackpoint><Time>2008-03-03T23:23:18Z</Time><Position><LatitudeDegrees>35.881438</LatitudeDegrees><LongitudeDegrees>-78.947490</LongitudeDegrees></Position><AltitudeMeters>78.004</AltitudeMeters><DistanceMeters>20825.445</DistanceMeters><Cadence>81</Cadence><Extensions><TPX xmlns=\"http://www.garmin.com/xmlschemas/ActivityExtension/v2\"><Watts>389</Watts></TPX></Extensions></Trackpoint><Trackpoint><Time>2008-03-03T23:23:19Z</Time><Position><LatitudeDegrees>35.881516</LatitudeDegrees><LongitudeDegrees>-78.947466</LongitudeDegrees></Position><AltitudeMeters>78.485</AltitudeMeters><DistanceMeters>20834.414</DistanceMeters><Cadence>83</Cadence><Extensions><TPX xmlns=\"http://www.garmin.com/xmlschemas/ActivityExtension/v2\"><Watts>431</Watts></TPX></Extensions></Trackpoint><Trackpoint><Time>2008-03-03T23:23:20Z</Time><Position><LatitudeDegrees>35.881596</LatitudeDegrees><LongitudeDegrees>-78.947442</LongitudeDegrees></Position><AltitudeMeters>78.485</AltitudeMeters><DistanceMeters>20843.631</DistanceMeters><Cadence>86</Cadence><Extensions><TPX xmlns=\"http://www.garmin.com/xmlschemas/ActivityExtension/v2\"><Watts>469</Watts></TPX></Extensions></Trackpoint><Trackpoint><Time>2008-03-03T23:23:21Z</Time><Position><LatitudeDegrees>35.881679</LatitudeDegrees><LongitudeDegrees>-78.947417</LongitudeDegrees></Position><AltitudeMeters>78.965</AltitudeMeters><DistanceMeters>20853.102</DistanceMeters><Cadence>89</Cadence><Extensions><TPX xmlns=\"http://www.garmin.com/xmlschemas/ActivityExtension/v2\"><Watts>490</Watts></TPX></Extensions></Trackpoint><Trackpoint><Time>2008-03-03T23:23:22Z</Time><Position><LatitudeDegrees>35.881765</LatitudeDegrees><LongitudeDegrees>-78.947393</LongitudeDegrees></Position><AltitudeMeters>79.446</AltitudeMeters><DistanceMeters>20862.875</DistanceMeters><Cadence>90</Cadence><Extensions><TPX xmlns=\"http://www.garmin.com/xmlschemas/ActivityExtension/v2\"><Watts>456</Watts></TPX></Extensions></Trackpoint><Trackpoint><Time>2008-03-03T23:23:23Z</Time><Position><LatitudeDegrees>35.881851</LatitudeDegrees><LongitudeDegrees>-78.947372</LongitudeDegrees></Position><AltitudeMeters>79.927</AltitudeMeters><DistanceMeters>20872.605</DistanceMeters><Cadence>90</Cadence><Extensions><TPX xmlns=\"http://www.garmin.com/xmlschemas/ActivityExtension/v2\"><Watts>449</Watts></TPX></Extensions></Trackpoint><Trackpoint><Time>2008-03-03T23:23:24Z</Time><Position><LatitudeDegrees>35.881935</LatitudeDegrees><LongitudeDegrees>-78.947350</LongitudeDegrees></Position><AltitudeMeters>80.407</AltitudeMeters><DistanceMeters>20882.154</DistanceMeters><Cadence>88</Cadence><Extensions><TPX xmlns=\"http://www.garmin.com/xmlschemas/ActivityExtension/v2\"><Watts>338</Watts></TPX></Extensions></Trackpoint><Trackpoint><Time>2008-03-03T23:23:25Z</Time><Position><LatitudeDegrees>35.882017</LatitudeDegrees><LongitudeDegrees>-78.947325</LongitudeDegrees></Position><AltitudeMeters>80.888</AltitudeMeters><DistanceMeters>20891.518</DistanceMeters><Cadence>86</Cadence><Extensions><TPX xmlns=\"http://www.garmin.com/xmlschemas/ActivityExtension/v2\"><Watts>212</Watts></TPX></Extensions></Trackpoint><Trackpoint><Time>2008-03-03T23:23:26Z</Time><Position><LatitudeDegrees>35.882097</LatitudeDegrees><LongitudeDegrees>-78.947300</LongitudeDegrees></Position><AltitudeMeters>80.888</AltitudeMeters><DistanceMeters>20900.666</DistanceMeters><Cadence>85</Cadence><Extensions><TPX xmlns=\"http://www.garmin.com/xmlschemas/ActivityExtension/v2\"><Watts>163</Watts></TPX></Ext
